vi "Destroy.vi"(8 "error in (no error)":errorcluster, 11 "Transceiver Thread":refnum<class "Transceiver Thread.lvclass">) -> (0 "error out":errorcluster, 3 "Transceiver Thread type":refnum<class "Transceiver Thread.lvclass">)   [LabVIEW 2021, in "DSF Core.lvlib" / "Transceiver Thread.lvclass"]
uses:
  Transceiver Thread.lvclass
  Transceiver Thread.lvclass/Transceiver Thread.ctl
  Transceiver/Transceiver.lvclass
  Buffer Converter/Buffer Converter.lvclass
  Plugin Thread.lvclass
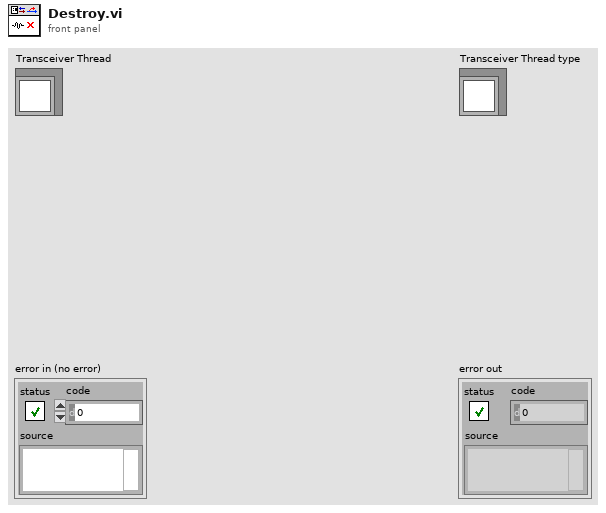
[diagram p1: front panel]
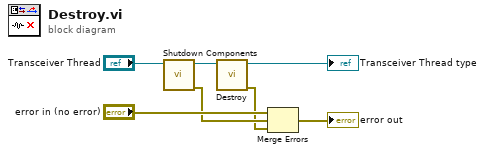
[diagram p0: block diagram]
diagram:
  n1 = call "Shutdown Components.vi"("Transceiver Thread in"="Transceiver Thread") -> ("error out"=w3:errorcluster, "Transceiver Thread out"=w5:refnum<class "Transceiver Thread.lvclass">)  [unwired: 9 in]
  n2 = call-parent "Destroy.vi"("Thread"=w5) -> ("error out"=w2:errorcluster, "Thread type"=→"Transceiver Thread type":refnum<class "Transceiver Thread.lvclass">)  [unwired: 9 in]
  n3 = Merge Errors("error in (no error)", w3, w2) -> (→"error out":errorcluster)
